vi "_create_hardware_items_and_aliases.vi"(8 "error in":errorcluster) -> (0 "error out":errorcluster, 4 "log":string)   [LabVIEW 2024]
uses:
  <vilib>/Plug-In SDKs/Clients/Metadata/Hardware Item.ctl
  <vilib>/Plug-In SDKs/Clients/Metadata/Extension.ctl
  <vilib>/Plug-In SDKs/Clients/Metadata Store V1/Metadata Store Client.lvlibp/API/Metadata Store V1/Create Hardware Item.vi
  <vilib>/Plug-In SDKs/Clients/Metadata Store V1/Metadata Store Client.lvlibp/API/Metadata Store V1/Create Alias (Metadata - Hardware Item).vi
  <vilib>/Plug-In SDKs/Clients/Metadata Store V1/Metadata Store Client.lvlibp
  <vilib>/Plug-In SDKs/Clients/Metadata/NI Metadata Types.lvlib
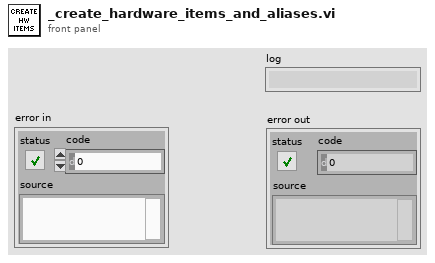
[diagram p1: front panel]
types:
  T1 = typedef "NI Metadata Types.lvlib/Hardware Item.ctl" = cluster{"model":string, "manufacturer":string, "part number":string, "serial number":string, "calibration due date":string, "asset identifier":string, "id":string, "link":string, "extensions":T2[], "schema id":string}
  T2 = typedef "NI Metadata Types.lvlib/Extension.ctl" = cluster{"name":string, "value":string}
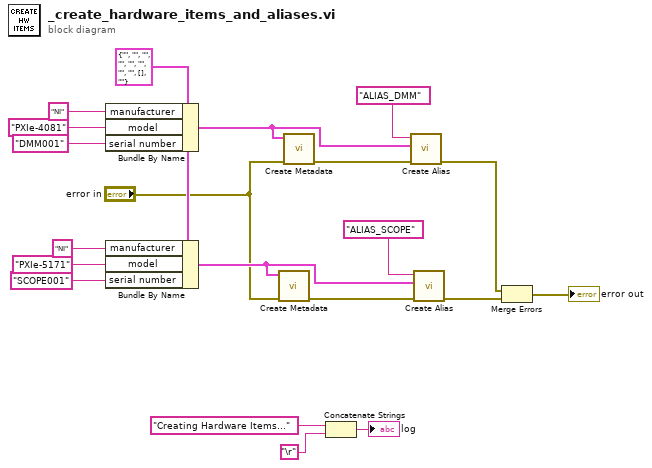
[diagram p0: block diagram]
diagram:
  w11 = T1 {"model"="", "manufacturer"="", "part number"="", "serial number"="", "calibration due date"="", "asset identifier"="", "id"="", "link"="", "extensions"=[], "schema id"=""} ("hardware item")
  n1 = Bundle By Name(cluster=w11, "manufacturer"="NI" ("operator name"), "model"="PXIe-4081" ("operator name"), "serial number"="DMM001") -> (w14:T1)
  n2 = Bundle By Name(cluster=w11, "manufacturer"="NI" ("operator name"), "model"="PXIe-5171", "serial number"="SCOPE001") -> (w17:T1)
  n3 = call-poly <vilib>:"Create Metadata.vi"("error in"="error in", "hardware item"=w17) -> ("error out"=w12:errorcluster)  [unwired: 8 in, 1 out]
  n4 = call-poly <vilib>:"Create Metadata.vi"("error in"="error in", "hardware item"=w14) -> ("error out"=w13:errorcluster)  [unwired: 8 in, 1 out]
  n5 = Concatenate Strings("Creating Hardware Items..." ("role"), "\r") -> (→"log":string)
  n6 = call-poly <vilib>:"Create Alias.vi"("error in"=w13, "hardware item"=w14, "alias name"="ALIAS_DMM") -> ("error out"=w18:errorcluster)  [unwired: 7 in, 1 out]
  n7 = call-poly <vilib>:"Create Alias.vi"("error in"=w12, "hardware item"=w17, "alias name"="ALIAS_SCOPE") -> ("error out"=w19:errorcluster)  [unwired: 7 in, 1 out]
  n8 = Merge Errors(w18, w19) -> (→"error out":errorcluster)
